vi "aqefwef.vi"() -> ()   [LabVIEW 2016]
panel:
  out "Vehicle.acc_pedal":u8
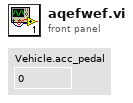
[diagram p1: front panel]
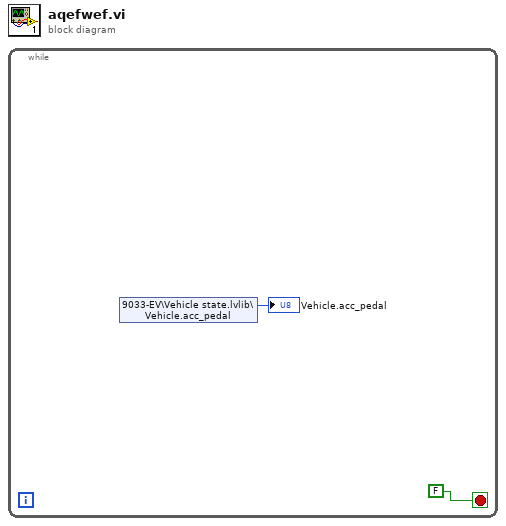
[diagram p0: block diagram]
diagram:
  n1 = while {
    stop <- FALSE stop-if-true
    n2 = shared-variable "9033-EV\\Vehicle state.lvlib\\Vehicle.acc_pedal"() -> (→"Vehicle.acc_pedal":u8)  [unwired: 1 in, 1 out]
  }
